vi "FindCloserAngle.vi"(9 "Central Angle":dbl, 10 "Angle 2":dbl, 11 "Angle 1":T1) -> (3 "Closer Angle":T1)   [LabVIEW 2011]
doc: "Given three angles - angle 1, angle 2, and \"central angle\", it finds which of angle 1 and angle 2 is closer to central angle."
uses:
  2 Typedefs/apparent wind direction.ctl
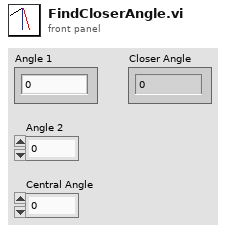
[diagram p1: front panel]
types:
  T1 = typedef "apparent wind direction.ctl" = dbl
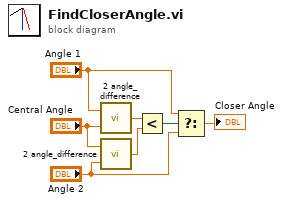
[diagram p0: block diagram]
diagram:
  n1 = call "2 angle_difference.vi"("Angle 2"="Central Angle", "Angle 1"="Angle 1") -> ("Difference"=w2:dbl)
  n2 = call "2 angle_difference.vi"("Angle 2"="Angle 2", "Angle 1"="Central Angle") -> ("Difference"=w1:dbl)
  n3 = Less?(x=w2, y=w1) -> (x < y?=w3:bool)
  n4 = Select(t="Angle 1", s=w3, f="Angle 2") -> (s? t:f=→"Closer Angle":T1)
